vi "Read detector calibrations.vi"(4 "Contrast B":sgl=40.0, 5 "Brightness B":sgl=40.0, 6 "Contrast A":sgl=26.0, 7 "Brightness A":sgl=40.0, 11 "Path":path) -> (3 "Latest 8-bit coefficients":sgl[][](array[numeric]))   [LabVIEW 2018]
uses:
  <vilib>/Utility/file.llb/Read From Spreadsheet File (string).vi
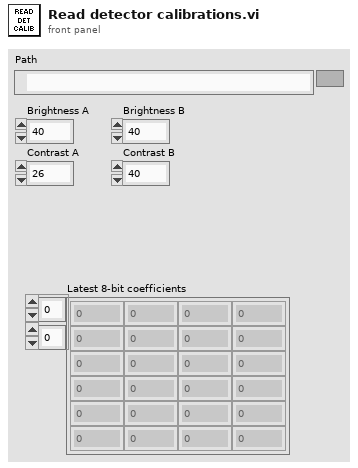
[diagram p1: front panel]
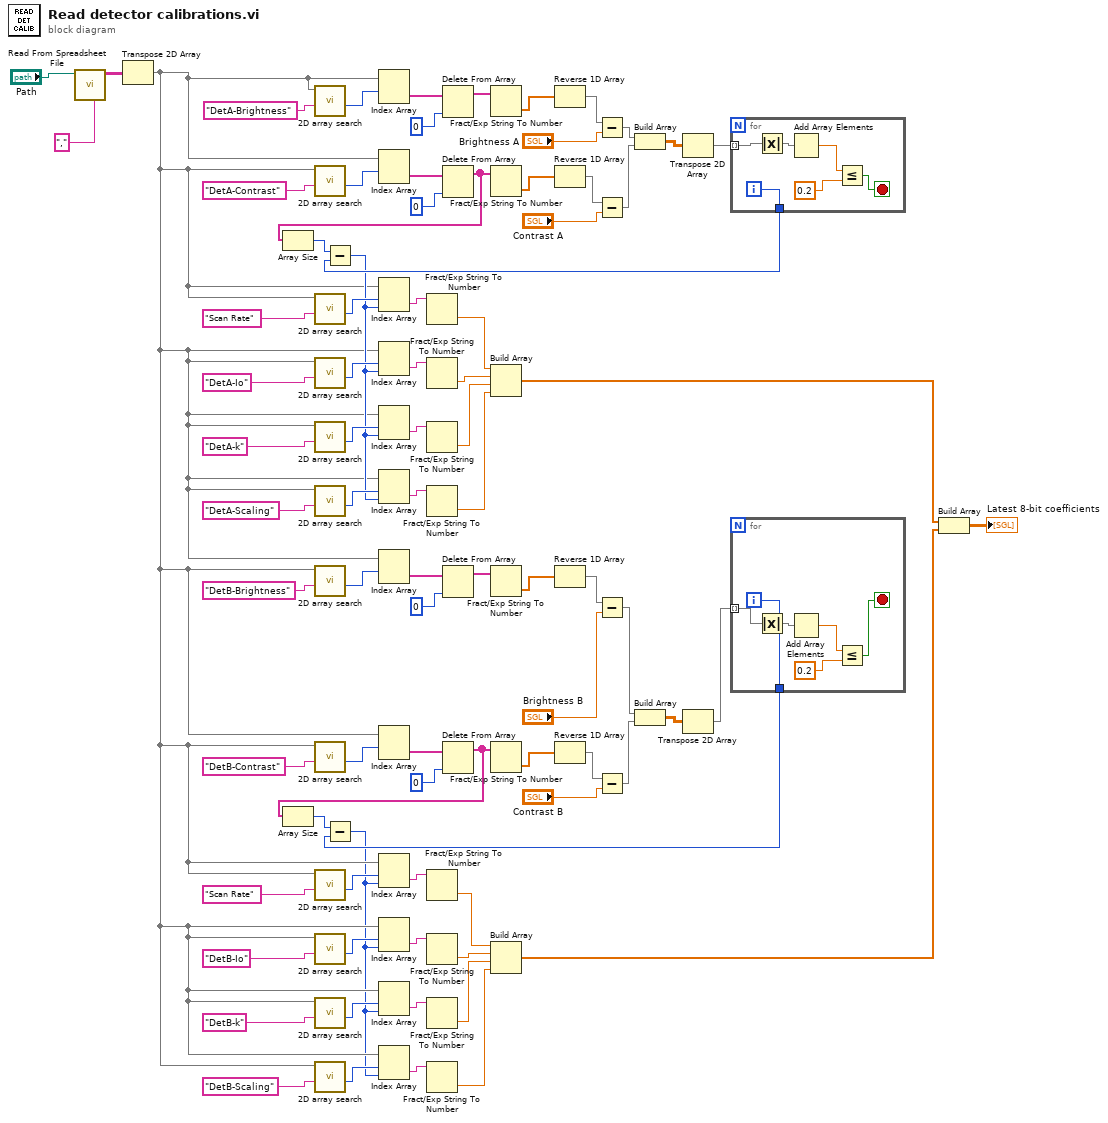
[diagram p0: block diagram]
diagram:
  n1 = call-poly <vilib>:"Read From Spreadsheet File.vi"("delimiter (\\t)"="," ("delimiter (\\t)"), "file path (dialog if empty)"="Path") -> ("all rows"=w82:string[][])  [unwired: 5 in, 4 out]
  n2 = Transpose 2D Array(2D array=w82) -> (transposed array=w3:string[][])
  n3 = call "2D array search.vi"("Search For"="DetA-Brightness", "Input Array"=w3) -> ("Row"=w83:i32)  [unwired: 7 in, 2 out]
  n4 = call "2D array search.vi"("Search For"="DetA-Contrast", "Input Array"=w3) -> ("Row"=w75:i32)  [unwired: 7 in, 2 out]
  n5 = call "2D array search.vi"("Search For"="Scan Rate", "Input Array"=w3) -> ("Row"=w19:i32)  [unwired: 7 in, 2 out]
  n6 = call "2D array search.vi"("Search For"="DetA-Io", "Input Array"=w3) -> ("Row"=w63:i32)  [unwired: 7 in, 2 out]
  n7 = call "2D array search.vi"("Search For"="DetA-k", "Input Array"=w3) -> ("Row"=w66:i32)  [unwired: 7 in, 2 out]
  n8 = call "2D array search.vi"("Search For"="DetA-Scaling", "Input Array"=w3) -> ("Row"=w9:i32)  [unwired: 7 in, 2 out]
  n9 = call "2D array search.vi"("Search For"="DetB-Brightness", "Input Array"=w3) -> ("Row"=w36:i32)  [unwired: 7 in, 2 out]
  n10 = call "2D array search.vi"("Search For"="DetB-Contrast", "Input Array"=w3) -> ("Row"=w44:i32)  [unwired: 7 in, 2 out]
  n11 = call "2D array search.vi"("Search For"="Scan Rate", "Input Array"=w3) -> ("Row"=w13:i32)  [unwired: 7 in, 2 out]
  n12 = call "2D array search.vi"("Search For"="DetB-Io", "Input Array"=w3) -> ("Row"=w54:i32)  [unwired: 7 in, 2 out]
  n13 = call "2D array search.vi"("Search For"="DetB-k", "Input Array"=w3) -> ("Row"=w51:i32)  [unwired: 7 in, 2 out]
  n14 = call "2D array search.vi"("Search For"="DetB-Scaling", "Input Array"=w3) -> ("Row"=w6:i32)  [unwired: 7 in, 2 out]
  n15 = Index Array(array=w3, index (row)=w83) -> (element=w80:string[])  [unwired: 1 in]
  n16 = Index Array(array=w3, index (row)=w75) -> (element=w26:string[])  [unwired: 1 in]
  n17 = Index Array(array=w3, index (row)=w36) -> (element=w38:string[])  [unwired: 1 in]
  n18 = Index Array(array=w3, index (row)=w44) -> (element=w42:string[])  [unwired: 1 in]
  n19 = Delete From Array(array=w80, index=0) -> (array with subset deleted=w78:string[])  [unwired: 1 in, 1 out]
  n20 = Delete From Array(array=w26, index=0) -> (array with subset deleted=w25:string[])  [unwired: 1 in, 1 out]
  n21 = Array Size(array=w25) -> (size(s)=w24:i32)
  n22 = Delete From Array(array=w38, index=0) -> (array with subset deleted=w40:string[])  [unwired: 1 in, 1 out]
  n23 = Delete From Array(array=w42, index=0) -> (array with subset deleted=w21:string[])  [unwired: 1 in, 1 out]
  n24 = Array Size(array=w21) -> (size(s)=w22:i32)
  n25 = Fract/Exp String To Number(string=w78) -> (number=w71:dbl[])  [unwired: 4 out]
  n26 = Fract/Exp String To Number(string=w25) -> (number=w72:dbl[])  [unwired: 4 out]
  n27 = Fract/Exp String To Number(string=w40) -> (number=w46:dbl[])  [unwired: 4 out]
  n28 = Fract/Exp String To Number(string=w21) -> (number=w45:dbl[])  [unwired: 4 out]
  n29 = Reverse 1D Array(array=w71) -> (reversed array=w30:dbl[])
  n30 = Reverse 1D Array(array=w72) -> (reversed array=w29:dbl[])
  n31 = Reverse 1D Array(array=w46) -> (reversed array=w28:dbl[])
  n32 = Reverse 1D Array(array=w45) -> (reversed array=w27:dbl[])
  n33 = Subtract(x=w30, y="Brightness A") -> (x-y=w67:dbl[])
  n34 = Subtract(x=w29, y="Contrast A") -> (x-y=w68:dbl[])
  n35 = Subtract(x=w28, y="Brightness B") -> (x-y=w50:dbl[])
  n36 = Subtract(x=w27, y="Contrast B") -> (x-y=w49:dbl[])
  n37 = Build Array(w67, w68) -> (w70:dbl[][])
  n38 = Build Array(w50, w49) -> (w47:dbl[][])
  n39 = Transpose 2D Array(2D array=w70) -> (transposed array=w69:dbl[][])
  n40 = Transpose 2D Array(2D array=w47) -> (transposed array=w48:dbl[][])
  n41 = for {
    tunnel: w69 -> [w91] mode=indexing
    tunnel: [w87] -> w23
    i -> [w87]
    stop <- w88 stop-if-true
    n42 = Absolute Value(x=w91) -> (abs(x)=w86:dbl[])
    n43 = Add Array Elements(numeric array=w86) -> (sum=w90:dbl)
    n44 = Less Or Equal?(x=w90, y=0.2) -> (x <= y?=w88:bool)
  }
  n45 = Subtract(x=w24, y=w23) -> (x-y=w7:i32)
  n46 = Index Array(array=w3, index (row)=w19, index (col)=w7) -> (element=w17:string)
  n47 = Index Array(array=w3, index (row)=w63, index (col)=w7) -> (element=w62:string)
  n48 = Index Array(array=w3, index (row)=w66, index (col)=w7) -> (element=w61:string)
  n49 = Index Array(array=w3, index (row)=w9, index (col)=w7) -> (element=w11:string)
  n50 = Fract/Exp String To Number(string=w17) -> (number=w16:dbl)  [unwired: 4 out]
  n51 = Fract/Exp String To Number(string=w62) -> (number=w60:dbl)  [unwired: 4 out]
  n52 = Fract/Exp String To Number(string=w61) -> (number=w59:dbl)  [unwired: 4 out]
  n53 = Fract/Exp String To Number(string=w11) -> (number=w8:dbl)  [unwired: 4 out]
  n54 = Build Array(w16, w60, w59, w8) -> (w33:dbl[])
  n55 = for {
    tunnel: w48 -> [w97] mode=indexing
    tunnel: [w93] -> w20
    i -> [w93]
    stop <- w94 stop-if-true
    n56 = Absolute Value(x=w97) -> (abs(x)=w92:dbl[])
    n57 = Add Array Elements(numeric array=w92) -> (sum=w96:dbl)
    n58 = Less Or Equal?(x=w96, y=0.2) -> (x <= y?=w94:bool)
  }
  n59 = Subtract(x=w22, y=w20) -> (x-y=w2:i32)
  n60 = Index Array(array=w3, index (row)=w13, index (col)=w2) -> (element=w15:string)
  n61 = Index Array(array=w3, index (row)=w54, index (col)=w2) -> (element=w55:string)
  n62 = Index Array(array=w3, index (row)=w51, index (col)=w2) -> (element=w56:string)
  n63 = Index Array(array=w3, index (row)=w6, index (col)=w2) -> (element=w4:string)
  n64 = Fract/Exp String To Number(string=w15) -> (number=w12:dbl)  [unwired: 4 out]
  n65 = Fract/Exp String To Number(string=w55) -> (number=w57:dbl)  [unwired: 4 out]
  n66 = Fract/Exp String To Number(string=w56) -> (number=w58:dbl)  [unwired: 4 out]
  n67 = Fract/Exp String To Number(string=w4) -> (number=w1:dbl)  [unwired: 4 out]
  n68 = Build Array(w12, w57, w58, w1) -> (w32:dbl[])
  n69 = Build Array(w33, w32) -> (→"Latest 8-bit coefficients":dbl[][])
